vi "RunOnce.vi"(1 "Instance":i32, 2 "Mode":enum16{"Reset", "Run"}(ring)) -> (0 "State":enum16{"RunOnce", "Finished"}(ring))   [LabVIEW 2013]
panel:
  out "InternalState":enum16{"RunOnce", "Finished"}[](array[ring])=[enum."RunOnce", enum."RunOnce", enum."RunOnce", enum."RunOnce", enum."RunOnce", enum."RunOnce", enum."RunOnce", enum."RunOnce", enum."RunOnce", enum."RunOnce"]
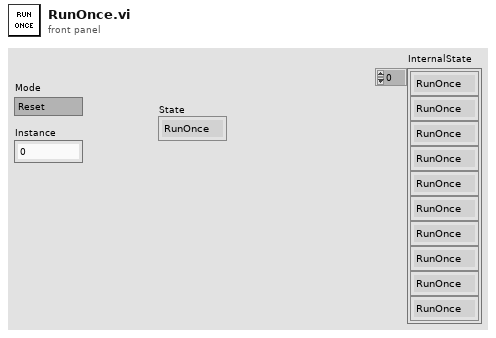
[diagram p1: front panel]
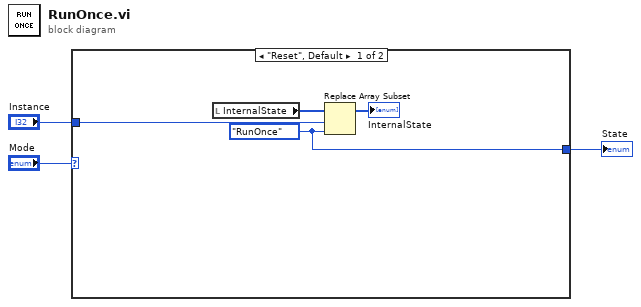
[diagram p0: block diagram]
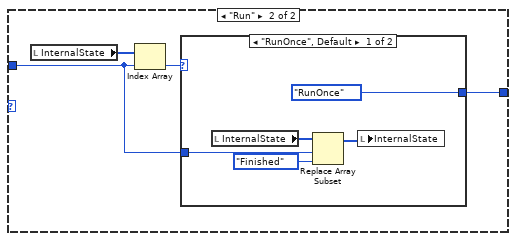
[diagram p2: hidden frame]
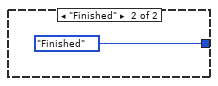
[diagram p3: hidden frame]
diagram:
  n1 = case shown="\"Reset\", Default" "Mode" {
    tunnel: [w4 w11] -> w1
    tunnel: "Instance" -> [w5 w8]
    frame "Reset", Default {
      w4 = enum16{"RunOnce", "Finished"}."RunOnce" ("State")
      n2 = local read "InternalState"() -> (w7:enum16{"RunOnce", "Finished"}[])
      n3 = Replace Array Subset(array=w7, new element=w4, index=w5) -> (→"InternalState":enum16{"RunOnce", "Finished"}[])
    }
    frame "Run" {
      n4 = local read "InternalState"() -> (w10:enum16{"RunOnce", "Finished"}[])
      n5 = Index Array(array=w10, index=w8) -> (element=w9:enum16{"RunOnce", "Finished"})
      n6 = case shown="\"RunOnce\", Default" w9 {
        tunnel: [enum16{"RunOnce", "Finished"}."RunOnce" ("State") enum16{"RunOnce", "Finished"}."Finished" ("State")] -> w11
        tunnel: w8 -> [w12 _]
        frame "RunOnce", Default {
          n7 = local read "InternalState"() -> (w14:enum16{"RunOnce", "Finished"}[])
          n8 = Replace Array Subset(array=w14, new element=enum16{"RunOnce", "Finished"}."Finished" ("State"), index=w12) -> (w15:enum16{"RunOnce", "Finished"}[])
          n9 = local write "InternalState"(w15) -> ()
        }
        frame "Finished" {
        }
      }
    }
  }
  "State" <- w1
